vi "Read Style.vi"(8 "error in (no error)":errorcluster, 11 "Splitter in":refnum<class "Splitter.lvclass">) -> (0 "error out":errorcluster, 2 "Splitter Style":T1 items=["Modern", "Classic", "System", "NXG"], 3 "Splitter out":refnum<class "Splitter.lvclass">)   [LabVIEW 2020, in "Splitter.lvclass"]
uses:
  Splitter.lvclass
  Splitter.lvclass/Splitter.ctl
  Typedefs/Splitter Style--Enum.ctl
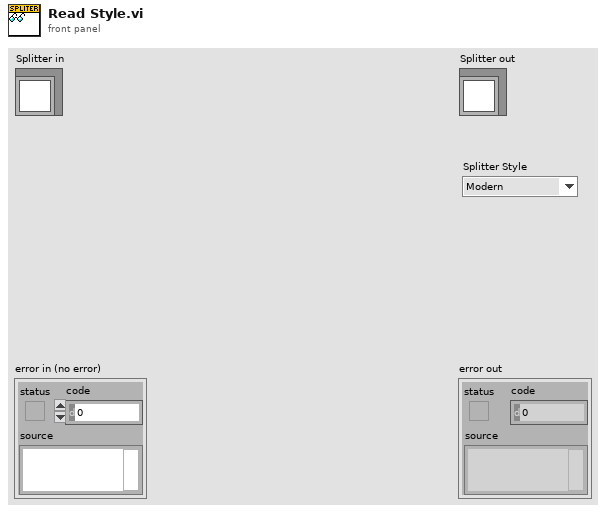
[diagram p1: front panel]
types:
  T1 = typedef "Splitter Style--Enum.ctl" = u16
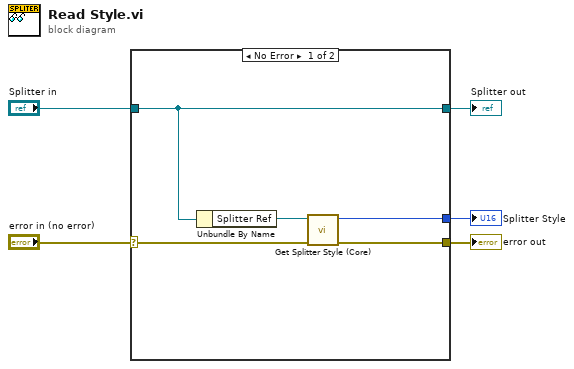
[diagram p0: block diagram]
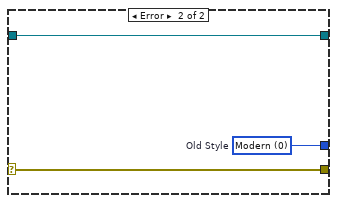
[diagram p2: hidden frame]
diagram:
  n1 = case shown="No Error" "error in (no error)" {
    selector: "error in (no error)" -> [w9 w13]
    tunnel: [w8 w13] -> w4
    tunnel: [w10 w12] -> w2
    tunnel: "Splitter in" -> [w10 w12]
    tunnel: [w7 w11] -> w1
    frame No Error {
      n2 = Unbundle By Name(w10) -> ("Splitter Ref"=w6:refnum<vi>)
      n3 = call "Get Splitter Style (Core).vi"("error in (no error)"=w9, "Splitter in"=w6) -> ("error out"=w8:errorcluster, "Old Style"=w7:T1)  [unwired: 6 in]
    }
    frame Error {
      w11 = T1 0 items=["Modern", "Classic", "System", "NXG"]  # Old Style
    }
  }
  "error out" <- w4
  "Splitter out" <- w2
  "Splitter Style" <- w1
